vi "Filter Contained Paths.vi"(2 "Output Array":path[](array[path])) -> (5 "Array":path[](array[path]))   [LabVIEW 2017]
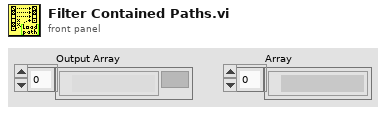
[diagram p1: front panel]
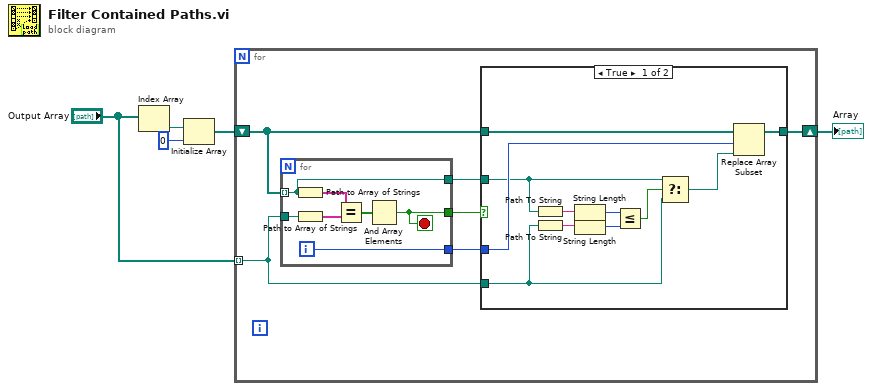
[diagram p0: block diagram]
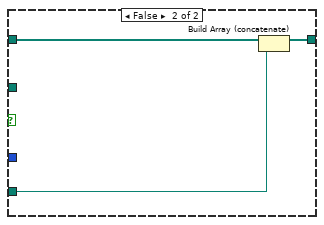
[diagram p2: hidden frame]
diagram:
  n1 = Index Array(array="Output Array") -> (element=w4:path)  [unwired: 1 in]
  n2 = Initialize Array(w4, 0 ("Dimension Size")) -> (w3:path[])
  n3 = for {
    tunnel: "Output Array" -> [w10] mode=indexing
    shift-right: [w11] -> w1
    shift-left: w3 -> [w9]
    n4 = for {
      tunnel: w10 -> [w15]
      tunnel: w9 -> [w13] mode=indexing
      tunnel: [w14] -> w8
      tunnel: [w13] -> w7
      tunnel: [w12] -> w6
      i -> [w12]
      stop <- w14 stop-if-true
      n5 = Path to Array of Strings(0:w13) -> (2:w17:string[])  [unwired: 1 out]
      n6 = Path to Array of Strings(0:w15) -> (2:w18:string[])  [unwired: 1 out]
      n7 = Equal?(x=w17, y=w18) -> (x = y?=w16:bool[])
      n8 = And Array Elements(Boolean array=w16) -> (logical AND=w14:bool)
    }
    n9 = case shown="True" w8 {
      tunnel: w10 -> [w24 w32]
      tunnel: [w28 w30] -> w11
      tunnel: w9 -> [w29 w31]
      tunnel: w7 -> [w25 _]
      tunnel: w6 -> [w26 _]
      frame True {
        n10 = Path To String(path=w25) -> (string=w22:string)
        n11 = Path To String(path=w24) -> (string=w23:string)
        n12 = String Length(string=w22) -> (length=w20:i32)
        n13 = String Length(string=w23) -> (length=w19:i32)
        n14 = Less Or Equal?(x=w20, y=w19) -> (x <= y?=w21:bool)
        n15 = Select(t=w25, s=w21, f=w24) -> (s? t:f=w27:path)
        n16 = Replace Array Subset(array=w29, new element=w27, index=w26) -> (w28:path[])
      }
      frame False {
        n17 = Build Array (concatenate)(w31, w32) -> (w30:path[])
      }
    }
  }
  "Array" <- w1
